vi "Flie Extention list.vi"(11 "file extention list IN":string[](array[string])) -> (3 "File extention list (out)":string[](array[string]))   [LabVIEW 2011]
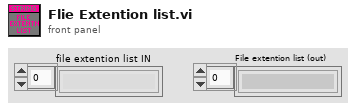
[diagram p1: front panel]
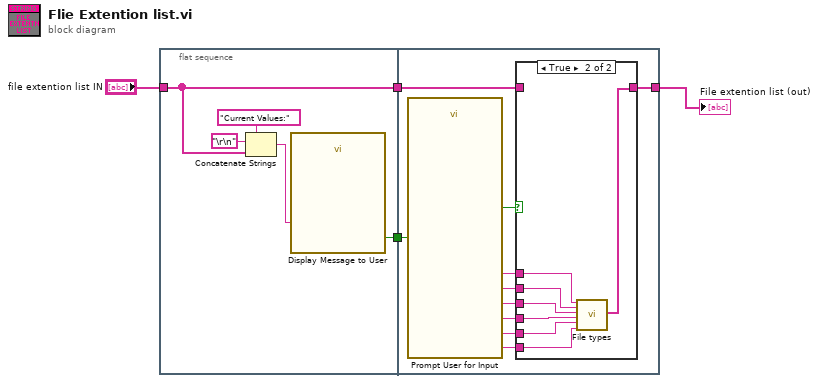
[diagram p0: block diagram]
diagram:
  n1 = flat-sequence {
    tunnel: "file extention list IN" -> [w6]
    tunnel: [w6] -> w4
    tunnel: [w9] -> w3
    tunnel: [w17] -> w2
    tunnel: w4 -> [w19]
    tunnel: w3 -> [w11]
    frame #0 {
      n2 = Concatenate Strings("Current Values:" ("string"), "\r\n", w6) -> (w5:string)
      n3 = call "Display Message to User"("Message"=w5) -> ("Change Values"=w9:bool)  [unwired: 9 in, 1 out]
    }
    frame #1 {
      n4 = call "Prompt User for Input"("Enable"=w11) -> ("6th File Type"=w10:string, "5th File Type"=w12:string, "4th File Type"=w13:string, "3rd File Type"=w14:string, "2nd File Type"=w15:string, "1st  file Type"=w16:string, "OK"=w18:bool)  [unwired: 11 in, 1 out]
      n5 = case shown="True" w18 {
        tunnel: w19 -> [w20 _]
        tunnel: [w20 w21] -> w17
        tunnel: w16 -> [_ w27]
        tunnel: w15 -> [_ w26]
        tunnel: w14 -> [_ w25]
        tunnel: w13 -> [_ w24]
        tunnel: w12 -> [_ w23]
        tunnel: w10 -> [_ w22]
        frame False {
        }
        frame True {
          n6 = call "File types.vi"("file type 1"=w27, "file type 2"=w26, "file type 3"=w25, "file type 4"=w24, "file type 5"=w23, "file type 6"=w22) -> ("Array"=w21:string[])  [unwired: 13 in]
        }
      }
    }
  }
  "File extention list (out)" <- w2
